vi "ex6-5.vi"   [LabVIEW 2013]
uses:
  <vilib>/NXT/Dual Mode Library/Sensors/EV3_Touch_Pressed.vi
  <vilib>/NXT/Dual Mode Library/Sensors/EV3_Infrared_Proxy.vi
  <vilib>/NXT/Dual Mode Library/Display/drawNumber.vi
  <vilib>/NXT/NXTIO Xnodes/NXTIONodeSubVIs/LEGOMoveAllMotors.vi
  <vilib>/NXT/Hardware/Plugins/Open Port/OpenPortAddress.ctl
  <vilib>/NXT/Subs/LVHSConnector.ctl
  <vilib>/NXT/NXTIO Xnodes/NXTIOXNode/NXTIO.xnode
  <vilib>/NXT/LegoClasses/BrickReference/BrickReference.lvclass
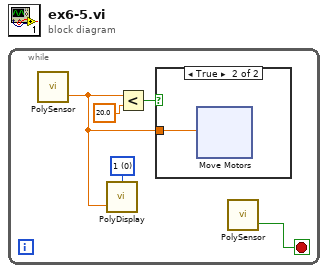
[diagram p0: block diagram]
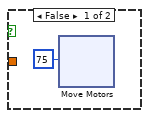
[diagram p2: hidden frame]
diagram:
  n1 = while {
    stop <- w2 stop-if-true
    w5 = i16 0 items=["1", "2", "3", "4", "5", "6", "7", "8", "9", "10", "11", "12"] ("Line")
    n2 = call-poly <vilib>:"PolySensor.vi"() -> ("Scaled Value"=w1:sgl)  [unwired: 3 in, 1 out]
    n3 = call-poly <vilib>:"PolyDisplay.vi"("number"=w1, "Line"=w5) -> ()  [unwired: 2 in, 1 out]
    n4 = Less?(x=w1, y=sgl 20.0) -> (x < y?=w3:bool)
    n5 = case shown="True" w3 {
      tunnel: w1 -> [_ w12]
      frame False {
        n6 = xnode "Move Motors"("Power/Speed 1"=i8 75) -> ()  [unwired: 2 in, 1 out]
      }
      frame True {
        n7 = xnode "Move Motors"("Power/Speed 1"=w12) -> ()  [unwired: 2 in, 1 out]
      }
    }
    n8 = call-poly <vilib>:"PolySensor.vi"() -> ("Pressed"=w2:bool)  [unwired: 3 in, 1 out]
  }
